vi "rsdc.vi"(2 "c":bool, 3 "d":bool, 4 "s":bool, 5 "r":bool) -> (0 "not q":bool, 1 "q":bool)   [LabVIEW 2017]
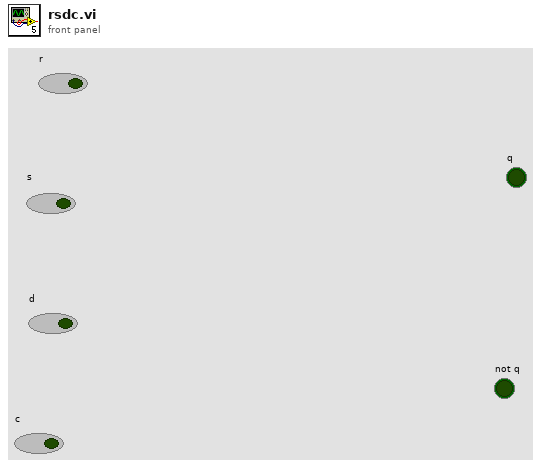
[diagram p1: front panel]
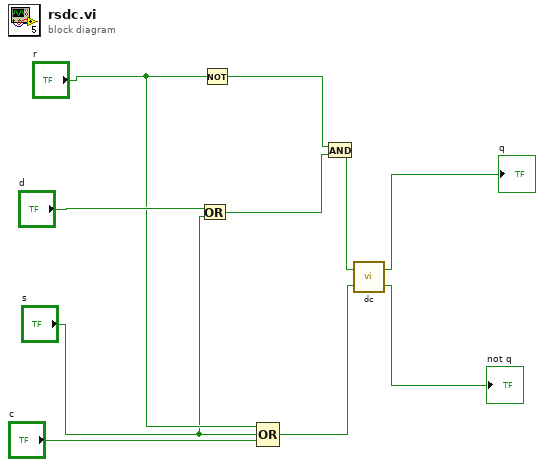
[diagram p0: block diagram]
diagram:
  n1 = Or(x="d", y="s") -> (x .or. y?=w5:bool)
  n2 = Not(x="r") -> (.not. x?=w6:bool)
  n3 = Compound Arithmetic op=OR("r", "s", "c") -> (w7:bool)
  n4 = And(x=w6, y=w5) -> (x .and. y?=w8:bool)
  n5 = call "dc.vi"("c"=w7, "d"=w8) -> ("not q"=→"not q":bool, "q"=→"q":bool)
